vi "EnFlo_Lab_Temp_Control.vi"() -> ()   [LabVIEW 2010]
uses:
  ADAM Client/Sub VIs/ADAM Controls/Update_scan_value.ctl
panel:
  out "EnFlo Lab:labstrat1:Av Temp":dbl
  out "EnFlo_Tunnel:Exit Duct:Dem Temp":dbl
  out "Reduction in air temp from ambient":dbl
  out "Approx Heat Extraction Value in kW":dbl
  out "EnFlo Lab:Desired:Air Temp":dbl
  out "Temperature Error":dbl
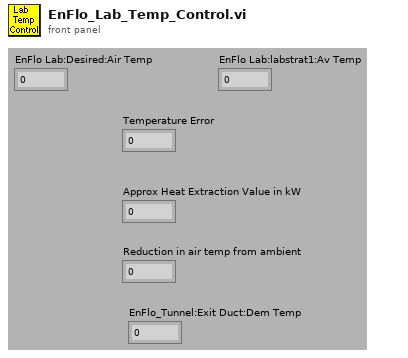
[diagram p1: front panel]
types:
  T1 = enum16{"Append to Global", "Read Global then Clear"}
  T2 = typedef "Update_scan_value.ctl" = cluster{"Channel Name":string, "New Value":dbl}
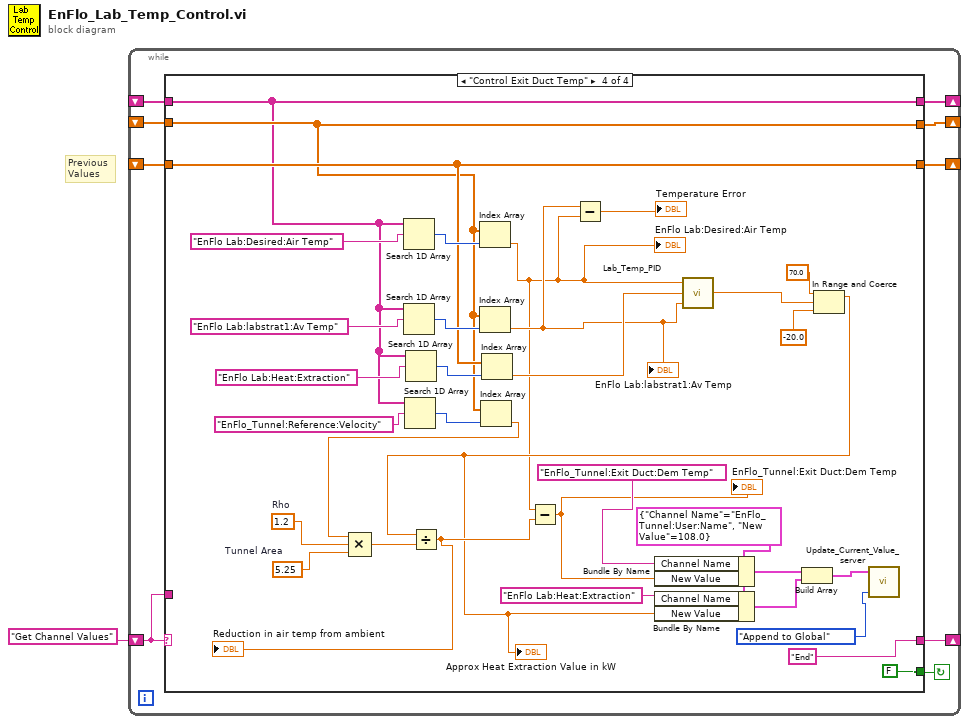
[diagram p0: block diagram]
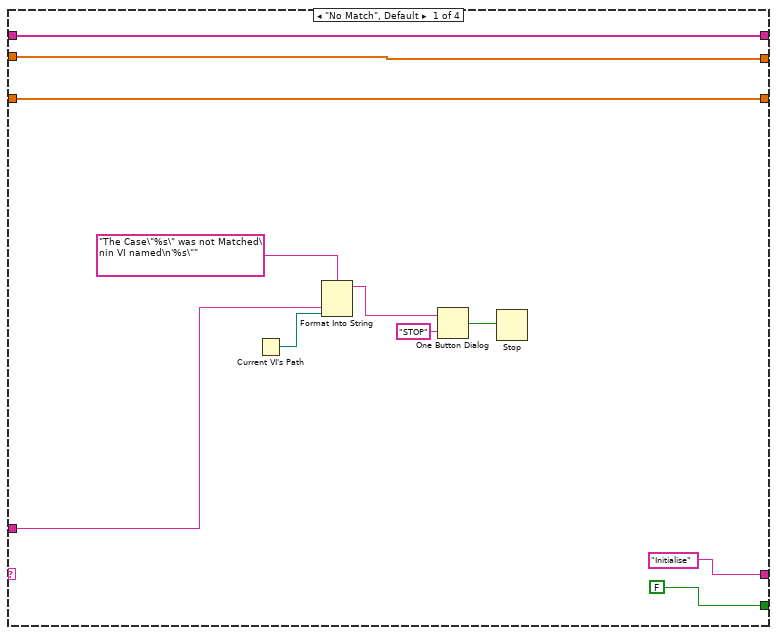
[diagram p2: hidden frame]
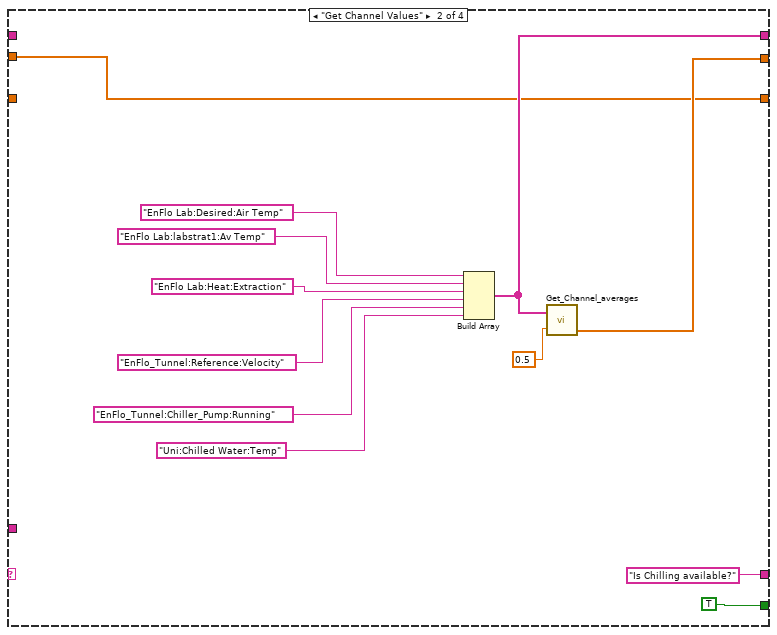
[diagram p3: hidden frame]
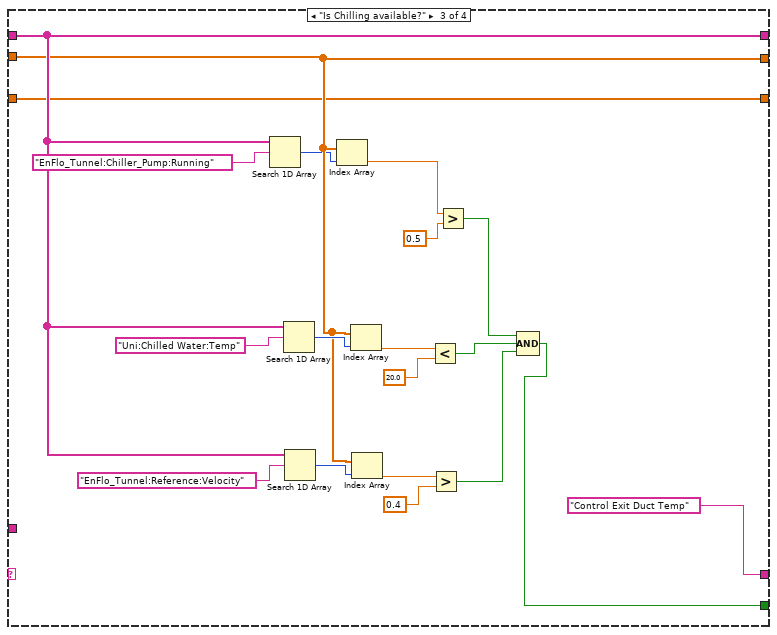
[diagram p4: hidden frame]
diagram:
  # "Previous\nValues"
  n1 = while {
    shift-left: "Get Channel Values" -> [w8]
    shift-right: [w9] -> _
    shift-right: [w6] -> _
    shift-left: _ -> [w4]
    shift-right: [w7] -> _
    shift-left: _ -> [w5]
    shift-right: [w3] -> _
    shift-left: _ -> [w2]
    stop <- w10 continue-if-true
    n2 = case shown="\"Control Exit Duct Temp\"" w8 {
      tunnel: [FALSE TRUE w34 FALSE] -> w10
      tunnel: ["Initialise" "Is Chilling available?" "Control Exit Duct Temp" "End"] -> w9
      tunnel: w8 -> [w16 _ _ _]
      tunnel: [w13 w25 w40 w75] -> w7
      tunnel: [w12 w24 w41 w74] -> w6
      tunnel: w5 -> [w13 w22 w40 w75]
      tunnel: w4 -> [w12 _ w41 w74]
      tunnel: [w11 w22 w39 w76] -> w3
      tunnel: w2 -> [w11 _ w39 w76]
      frame "No Match", Default {
        n3 = Current VI's Path() -> (path=w15:path)
        n4 = Format Into String(format string="The Case\"%s\" was not Matched\nin VI named\n'%s\"" ("Format String"), w16, w15) -> (resulting string=w19:string)  [unwired: 2 in, 1 out]
        n5 = One Button Dialog(message=w19, button name ("OK")="STOP") -> (true=w17:bool)
        n6 = Stop(stop? (T)=w17) -> ()
      }
      frame "Get Channel Values" {
        n7 = Build Array("EnFlo Lab:Desired:Air Temp", "EnFlo Lab:labstrat1:Av Temp", "EnFlo Lab:Heat:Extraction", "EnFlo_Tunnel:Reference:Velocity", "EnFlo_Tunnel:Chiller_Pump:Running", "Uni:Chilled Water:Temp") -> (w24:string[])
        n8 = call "Get_Channel_averages.vi"("Desired Ch Names"=w24, "Averaging time (mins)"=0.5) -> ("number"=w25:dbl[])  [unwired: 1 in, 2 out]
      }
      frame "Is Chilling available?" {
        n9 = Search 1D Array(1D array=w41, element="EnFlo_Tunnel:Chiller_Pump:Running") -> (index of element=w38:i32)  [unwired: 1 out]
        n10 = Search 1D Array(1D array=w41, element="Uni:Chilled Water:Temp") -> (index of element=w51:i32)  [unwired: 1 out]
        n11 = Search 1D Array(1D array=w41, element="EnFlo_Tunnel:Reference:Velocity") -> (index of element=w46:i32)  [unwired: 1 out]
        n12 = Index Array(array=w40, index=w38) -> (element=w35:dbl)
        n13 = Index Array(array=w40, index=w51) -> (element=w50:dbl)
        n14 = Index Array(array=w40, index=w46) -> (element=w47:dbl)
        n15 = Less?(x=w50, y=20.0) -> (x < y?=w44:bool)
        n16 = Greater?(x=w47, y=0.4) -> (0:w43:bool)
        n17 = Greater?(x=w35, y=0.5) -> (0:w36:bool)
        n18 = Compound Arithmetic op=AND(w36, w44, w43) -> (w34:bool)
      }
      frame "Control Exit Duct Temp" {
        w58 = T2 {"Channel Name"="EnFlo_Tunnel:User:Name", "New Value"=108.0} ("Update Scan Value Cluster")
        w71 = 5.25  # Tunnel Area
        w72 = 1.2  # Rho
        n19 = Search 1D Array(1D array=w74, element="EnFlo Lab:Desired:Air Temp") -> (index of element=w87:i32)  [unwired: 1 out]
        n20 = Search 1D Array(1D array=w74, element="EnFlo Lab:labstrat1:Av Temp") -> (index of element=w83:i32)  [unwired: 1 out]
        n21 = Search 1D Array(1D array=w74, element="EnFlo_Tunnel:Reference:Velocity") -> (index of element=w77:i32)  [unwired: 1 out]
        n22 = Search 1D Array(1D array=w74, element="EnFlo Lab:Heat:Extraction") -> (index of element=w82:i32)  [unwired: 1 out]
        n23 = Index Array(array=w75, index=w87) -> (element=w54:dbl)
        "EnFlo Lab:Desired:Air Temp" <- w54
        n24 = Index Array(array=w75, index=w83) -> (element=w56:dbl)
        "EnFlo Lab:labstrat1:Av Temp" <- w56
        n25 = Index Array(array=w75, index=w77) -> (element=w73:dbl)
        n26 = Compound Arithmetic op=MULTIPLY(w73, w72, w71) -> (w70:dbl)
        n27 = Index Array(array=w76, index=w82) -> (element=w81:dbl)
        n28 = Subtract(x=w56, y=w54) -> (x-y=→"Temperature Error":dbl)
        n29 = call "Lab_Temp_PID.vi"("Present Value"=w56, "Previous Control Sum"=w81, "Setpoint"=w54) -> ("Dem Output"=w57:dbl)
        n30 = In Range and Coerce(upper limit=70.0, x=w57, lower limit=-20.0) -> (coerced(x)=w60:dbl)  [unwired: 1 out]
        "Approx Heat Extraction Value in kW" <- w60
        n31 = Divide(x=w60, y=w70) -> (x/y=w69:dbl)
        "Reduction in air temp from ambient" <- w69
        n32 = Subtract(x=w54, y=w69) -> (x-y=w65:dbl)
        "EnFlo_Tunnel:Exit Duct:Dem Temp" <- w65
        n33 = Bundle By Name(cluster=w58, "Channel Name"="EnFlo_Tunnel:Exit Duct:Dem Temp", "New Value"=w65) -> (w62:T2)
        n34 = Bundle By Name(cluster=w58, "Channel Name"="EnFlo Lab:Heat:Extraction", "New Value"=w60) -> (w59:T2)
        n35 = Build Array(w62, w59) -> (w67:T2[])
        n36 = call "Update_Current_Value_server.vi"("Mode"=T1."Append to Global", "Update array in"=w67) -> ()  [unwired: 1 in, 1 out]
      }
    }
  }
